vi "Polyphase Filter_Filter (SGL).vi"(0 "X":sgl[](array[numeric]), 1 "output phase in":i32, 2 "init? (F)":bool, 5 "FIR Coefficients":sgl[](array[numeric]), 7 "factor":T2, 9 "skip point in":i32, 11 "mode":T1 items=["Default"=-1, "No Rate Change"=0, "Interpolation"=1, "Decimation"=2, "Rational"=3], 12 "State in":sgl[](array[numeric]), 13 "zero phase? (T)":bool) -> (3 "output phase out":i32, 4 "Filtered X":sgl[](array[numeric]), 10 "skip point out":i32, 14 "State out":sgl[](array[numeric]), 15 "error":i32)   [LabVIEW 2020, in "NI_AAL_Filter.lvlib"]
uses:
  <vilib>/Analysis/NI_AAL_Filter.lvlib
  <vilib>/Analysis/3filter.llb/Polyphase Filter_Factor.ctl
  <vilib>/Analysis/3filter.llb/Polyphase Filter_Mode.ctl
  <resource>/lvanlys.dll
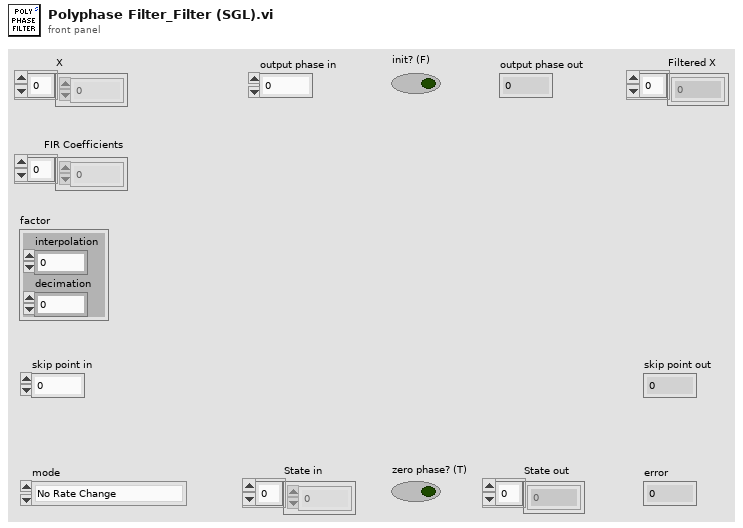
[diagram p1: front panel]
types:
  T1 = typedef "NI_AAL_Filter.lvlib/Polyphase Filter_Mode.ctl" = i32
  T2 = typedef "NI_AAL_Filter.lvlib/Polyphase Filter_Factor.ctl" = cluster{"interpolation":i32, "decimation":i32}
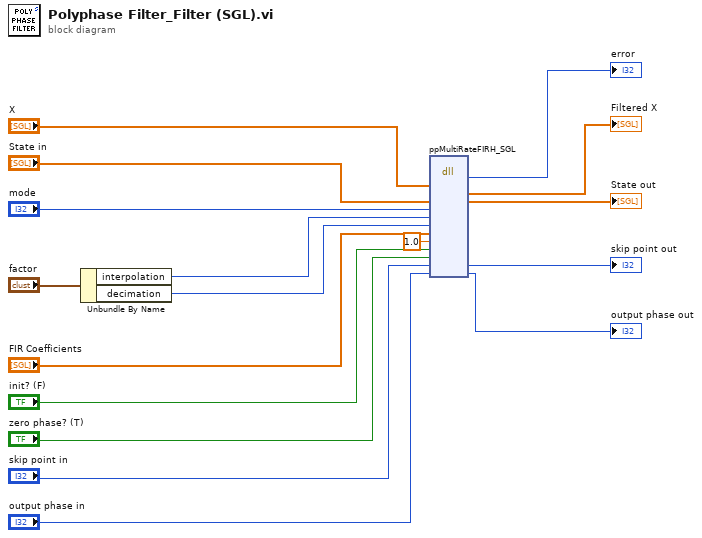
[diagram p0: block diagram]
diagram:
  n1 = Unbundle By Name("factor") -> ("interpolation"=w8:i32, "decimation"=w7:i32)
  n2 = dll-call lib="e:/builds/penguin/labview/branches/2020/dev/dist/resource/lvanlys.*" fn="ppMultiRateFIRH_SGL" ("LVDFD.dll:MRateFIRH")("inputDataH"="X", "initialStatesH"="State in", "filterMode"="mode", "Lfactor"=w8, "Mfactor"=w7, "coefH"="FIR Coefficients", "gain"=sgl 1.0 ("gainH"), "init"="init? (F)", "zeroPhase"="zero phase? (T)", "skipPoint"="skip point in", "outputPhase"="output phase in") -> ("return type"=→"error":i32, "outputDataH"=→"Filtered X":sgl[], "initialStatesH"=→"State out":sgl[], "skipPoint"=→"skip point out":i32, "outputPhase"=→"output phase out":i32)  [unwired: 11 in, 3 out]
